vi "Destroy.vi"(8 "Error In":errorcluster, 11 "reference in":refnum<class "VdDigitalControl_AdvantechADAM.lvclass">) -> (0 "Error Out":errorcluster, 3 "reference out":refnum<class "VdDigitalControl_AdvantechADAM.lvclass">)   [LabVIEW 2020, in "VdDigitalControl_AdvantechADAM.lvclass"]
uses:
  VdDigitalControl_AdvantechADAM.lvclass
  VdDigitalControl_AdvantechADAM.lvclass/VdDigitalControl_AdvantechADAM.ctl
  VdDigitalControl_class/VdDigitalControl.lvclass
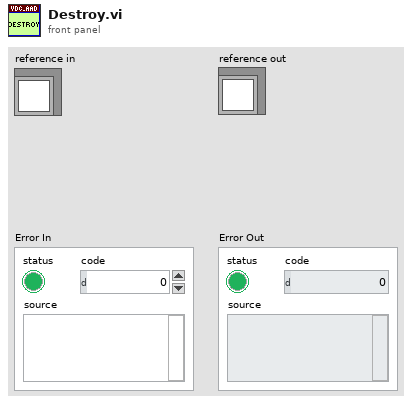
[diagram p1: front panel]
types:
  T1 = typedef "VdDigitalControl_AdvantechADAM.lvclass/ObjectAttributes.ctl" = cluster{"VISARef":refnum<visa-resource-name>}
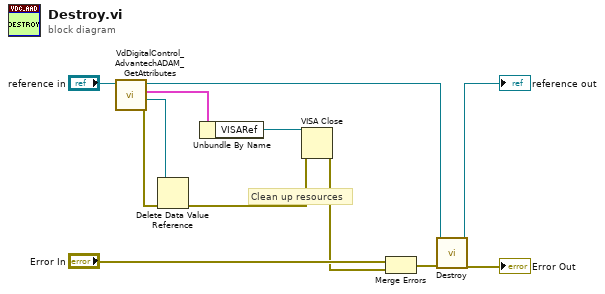
[diagram p0: block diagram]
diagram:
  # "Clean up resources"
  n1 = call "VdDigitalControl_AdvantechADAM_GetAttributes.vi"("reference in"="reference in") -> ("error out"=w10:errorcluster, "DataRef"=w7:refnum<data-value>, "Data"=w9:T1, "reference out"=w8:refnum<class "VdDigitalControl_AdvantechADAM.lvclass">)  [unwired: 7 in]
  n2 = Delete Data Value Reference(data value reference=w7, error in=w10) -> (error out=w2:errorcluster)  [unwired: 1 out]
  n3 = Unbundle By Name(w9) -> ("VISARef"=w3:refnum<visa-resource-name>)
  n4 = VISA Close(VISA resource name=w3, error in (no error)=w2) -> (error out=w1:errorcluster)
  n5 = Merge Errors("Error In", w1) -> (w12:errorcluster)
  n6 = call-parent "Destroy.vi"("Error In"=w12, "reference in"=w8) -> ("Error Out"=→"Error Out":errorcluster, "reference out"=→"reference out":refnum<class "VdDigitalControl_AdvantechADAM.lvclass">)  [unwired: 8 in]
